vi "PH_BL-Master.set modified data.vi"(0 "i ref in":refnum<vi>, 2 "i attribute":T1={"Remote controlled"=FALSE, "Boolean Condition Service Subscriber"=[], "Picture Condition Service Subscriber"=[], "R2S"={"GUI Ref"=refnum, "State"=FALSE}, "Vacua"=[], "O2 Inspection"=[], "Boolean Status Service Subscriber"=[], "Picture Status Service Subscriber"=[], "6P 4Q Service Subscriber"=[], "Index of latest 6P 4Q changing Instance"=-1, "Index of latest Picture Status changing Instance"=-1, "Index of latest Boolean Status changing Instance"=-1, "Vision ID on same Node"="N/A", "Start Phase over?"=FALSE, "GUI Ref Delete"=refnum} {"6P 4Q Service Subscriber"."Selector" items=["unknown", "Position I", "Position II", "Position III", "Position IV", "moving"]; "Picture Status Service Subscriber"."Status" items=["no info", "off/false/out", "on/true/in", "Failure", "Alarm", "Status 1", "Status 2", "Status 3"]; "Boolean Status Service Subscriber"."Status" items=["no info", "off/false/out", "on/true/in", "Failure", "Alarm", "Status 1", "Status 2", "Status 3"]; "O2 Inspection"."State" items=["no info", "off/false/out", "on/true/in", "Failure", "Alarm", "Status 1", "Status 2", "Status 3"]}, 5 "error in (no error)":errorcluster) -> (14 "i ref out":refnum<vi>, 19 "error out":errorcluster)   [LabVIEW 2014, in "PH_BL-Master.lvlib"]
doc: "Writes the data into the attribute of an object. Then, the attribute dara are unlocked using the \"release\" method. Prior to calling THIS method, the attribute data must have been locked using the methods \"lock\" or \"get data to modify\".\n\n\nLicense Agreement for this software:\n\nCopyright (C)\nGesellschaft für Schwerionenforschung, GSI\nPlanckstr. 1\n64291 Darmstadt\nGermany\n\nContact: D.Beck@gsi.de \n\nThis program is free software; you can redistribute it and/or modify it under the terms of the GNU General Public License as published by the Free Software Foundation; either version 2 of the license, or (at your option) any later version.\n\nThis program is distributed in the hope that it will be useful, but WITHOUT ANY WARRANTY; without even the implied warranty of MERCHANTABILITY or FITNESS FOR A PARTICULAR PURPOSE. See the GNU General License for more details (http://www.gnu.org).\n\nGesellschaft für Schwerionenforschung, GSI\nPlanckstr. 1, 64291 Darmstadt, Germany\nFor all questions and ideas contact: M.Richter@gsi.de, H.Brand@gsi.de or D.Beck@gsi.de.\nLast update: 17-JUN-2004"
uses:
  PH_BL-Master.lvlib
  PH_BL-Master.i attribute.ctl
  PH_Basics/PH_StatusHandler/PH_StatusHandler.Status.ctl
  PH_BL-Master.Status Subscriber Class.ctl
  PH_Motion/PH_4_Pos_Selector/PH_4_Pos_Selector.Position Selector.ctl
  CS_Core/CSObj/CSObj.lvlib
  PH_Basics/PH_StatusHandler/PH_StatusHandler.lvlib
  PH_Motion/PH_4_Pos_Selector/PH_4_Pos_Selector.lvlib
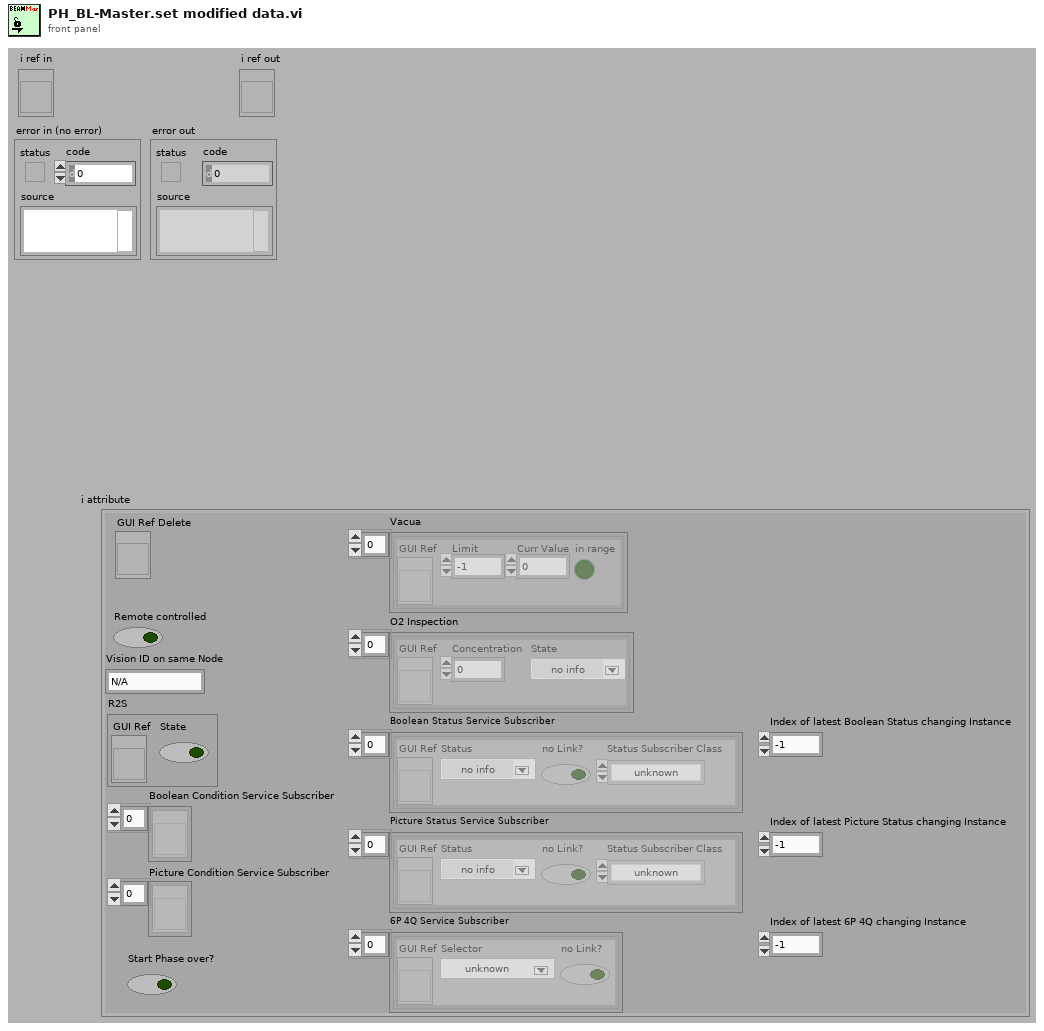
[diagram p1: front panel]
types:
  T1 = typedef "PH_BL-Master.lvlib/PH_BL-Master.i attribute.ctl" = cluster{"Remote controlled":bool, "Boolean Condition Service Subscriber":refnum<vi>[], "Picture Condition Service Subscriber":refnum<vi>[], "R2S":cluster{"GUI Ref":refnum<vi>, "State":bool}, "Vacua":cluster{"GUI Ref":refnum<vi>, "Limit":dbl, "Curr Value":dbl, "in range":bool}[], "O2 Inspection":cluster{"GUI Ref":refnum<vi>, "Concentration":dbl, "State":T2}[], "Boolean Status Service Subscriber":cluster{"GUI Ref":refnum<vi>, "Status":T2, "no Link?":bool, "Status Subscriber Class":T3}[], "Picture Status Service Subscriber":cluster{"GUI Ref":refnum<vi>, "Status":T2, "no Link?":bool, "Status Subscriber Class":T3}[], "6P 4Q Service Subscriber":cluster{"GUI Ref":refnum<vi>, "Selector":T4, "no Link?":bool}[], "Index of latest 6P 4Q changing Instance":i32, "Index of latest Picture Status changing Instance":i32, "Index of latest Boolean Status changing Instance":i32, "Vision ID on same Node":string, "Start Phase over?":bool, "GUI Ref Delete":refnum<vi>}
  T2 = typedef "PH_StatusHandler.lvlib/PH_StatusHandler.Status.ctl" = i16
  T3 = typedef "PH_BL-Master.lvlib/PH_BL-Master.Status Subscriber Class.ctl" = enum16{"unknown", "Switch", "BB", "6P Switch", "Switch GUI", "Switch and 6P State", "Force Sensor"}
  T4 = typedef "PH_4_Pos_Selector.lvlib/PH_4_Pos_Selector.Position Selector.ctl" = u16
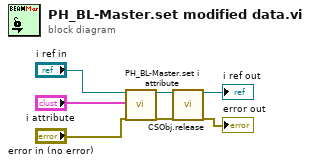
[diagram p0: block diagram]
diagram:
  n1 = call "PH_BL-Master.set i attribute.vi"("i ref in"="i ref in", "i attribute"="i attribute", "error in (no error)"="error in (no error)") -> ("i ref out"=w4:refnum<vi>, "error out"=w3:errorcluster)  [unwired: 15 in]
  n2 = call "CSObj.release.vi"("i ref in"=w4, "error in (no error)"=w3) -> ("i ref out"=→"i ref out":refnum<vi>, "error out"=→"error out":errorcluster)  [unwired: 16 in]
